vi "Filter and Sort Items.vi"(5 "Sort Info":T5={"Sort Column"=enum."Description", "Ascending?"=FALSE, "Enabled?"=FALSE}, 7 "Filter Info":T7={"Filter Column"=enum."Description", "Filter Type"=enum."Contains", "Filter Value"="", "New Data?"=FALSE, "Enabled?"=FALSE}, 8 "error in (no error)":errorcluster, 10 "New VI Data":T1[](array[typedef]), 11 "Saved VI Data":T1[](array[typedef])) -> (0 "error out":errorcluster, 1 "Displayed Indices":i32[](array[numeric]), 2 "New VI Data out":T1[](array[typedef]), 3 "Saved VI Data out":T1[](array[typedef]))   [LabVIEW 2020, in "VI Properties Editor.lvlib"]
doc: "Filters <B>Saved VI Data</B> according to <B>Filter</B>."
uses:
  VI Properties Editor.lvlib
  <vilib>/regexp/Match Regular Expression.xnode
  <vilib>/picture/picture.llb/imagedata.ctl
  CTLs/VI Properties.ctl
  CTLs/Control Properties.ctl
  CTLs/VI Data.ctl
  CTLs/Column Name.ctl
  CTLs/Filter Type.ctl
  CTLs/Filter Info.ctl
  CTLs/Sort Info.ctl
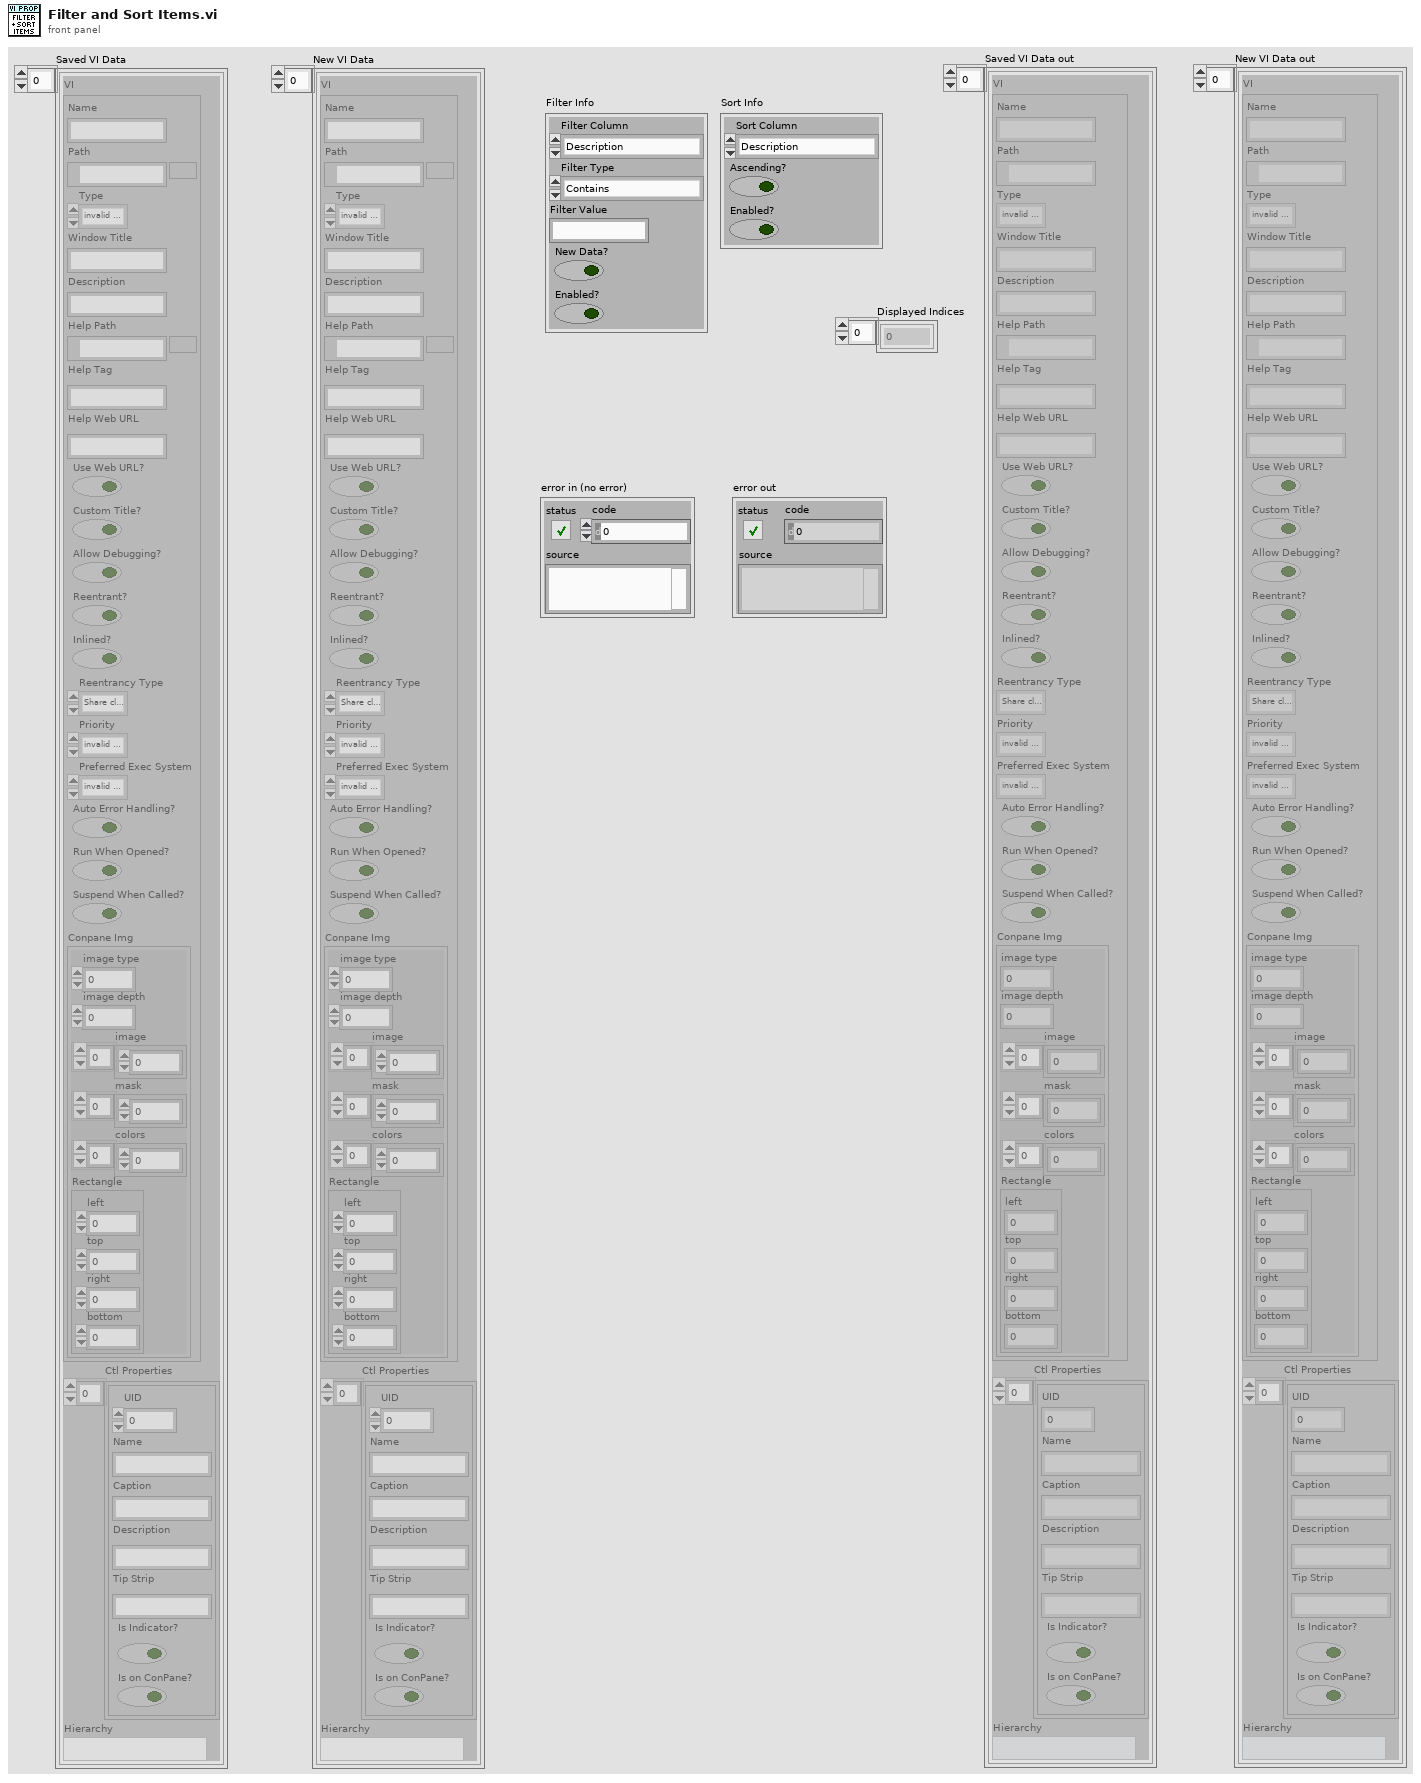
[diagram p1: front panel]
types:
  T1 = typedef "VI Properties Editor.lvlib/VI Data.ctl" = cluster{"VI":T2, "Ctl Properties":T4[], "Hierarchy":string}
  T2 = typedef "VI Properties Editor.lvlib/VI Properties.ctl" = cluster{"Name":string, "Path":path, "Type":enum32{"invalid VI type", "Standard VI", "Control VI", "Global VI", "Polymorphic VI", "Configuration VI", "SubSystem", "Facade VI", "Method VI", "Statechart Diagram VI"}, "Window Title":string, "Description":string, "Help Path":path, "Help Tag":string, "Help Web URL":string, "Use Web URL?":bool, "Custom Title?":bool, "Allow Debugging?":bool, "Reentrant?":bool, "Inlined?":bool, "Reentrancy Type":enum16{"Share clones between instances", "Preallocate clone for each instance"}, "Priority":enum32{"invalid priority", "background priority", "normal priority", "above normal priority", "high priority", "time critical priority", "subroutine"}, "Preferred Exec System":enum32{"invalid execution system", "user interface", "standard", "instrument i/o", "data acquisition", "other 1", "other 2", "same as caller"}, "Auto Error Handling?":bool, "Run When Opened?":bool, "Suspend When Called?":bool, "Conpane Img":T3}
  T3 = typedef "imagedata.ctl" = cluster{"image type":i32, "image depth":i32, "image":u8[], "mask":u8[], "colors":u32[], "Rectangle":cluster{"left":i16, "top":i16, "right":i16, "bottom":i16}}
  T4 = typedef "VI Properties Editor.lvlib/Control Properties.ctl" = cluster{"UID":i32, "Name":string, "Caption":string, "Description":string, "Tip Strip":string, "Is Indicator?":bool, "Is on ConPane?":bool}
  T5 = typedef "VI Properties Editor.lvlib/Sort Info.ctl" = cluster{"Sort Column":T6, "Ascending?":bool, "Enabled?":bool}
  T6 = typedef "VI Properties Editor.lvlib/Column Name.ctl" = enum16{"Name", "Path", "Type", "Window Title", "Description", "Help Path", "Help Tag", "Custom Title?", "Reentrancy", "Inlined?", "Help URL", "Help Type", "Allow Debugging?", "Auto Error Handling?", "Run When Opened?", "Suspend When Called?", "Priority", "Preferred Exec Sytem"}
  T7 = typedef "VI Properties Editor.lvlib/Filter Info.ctl" = cluster{"Filter Column":T6, "Filter Type":T8, "Filter Value":string, "New Data?":bool, "Enabled?":bool}
  T8 = typedef "VI Properties Editor.lvlib/Filter Type.ctl" = enum16{"Contains", "Equals", "Starts with", "Ends with", "Does not contain", "Does not equal", "Is empty", "Is not empty"}
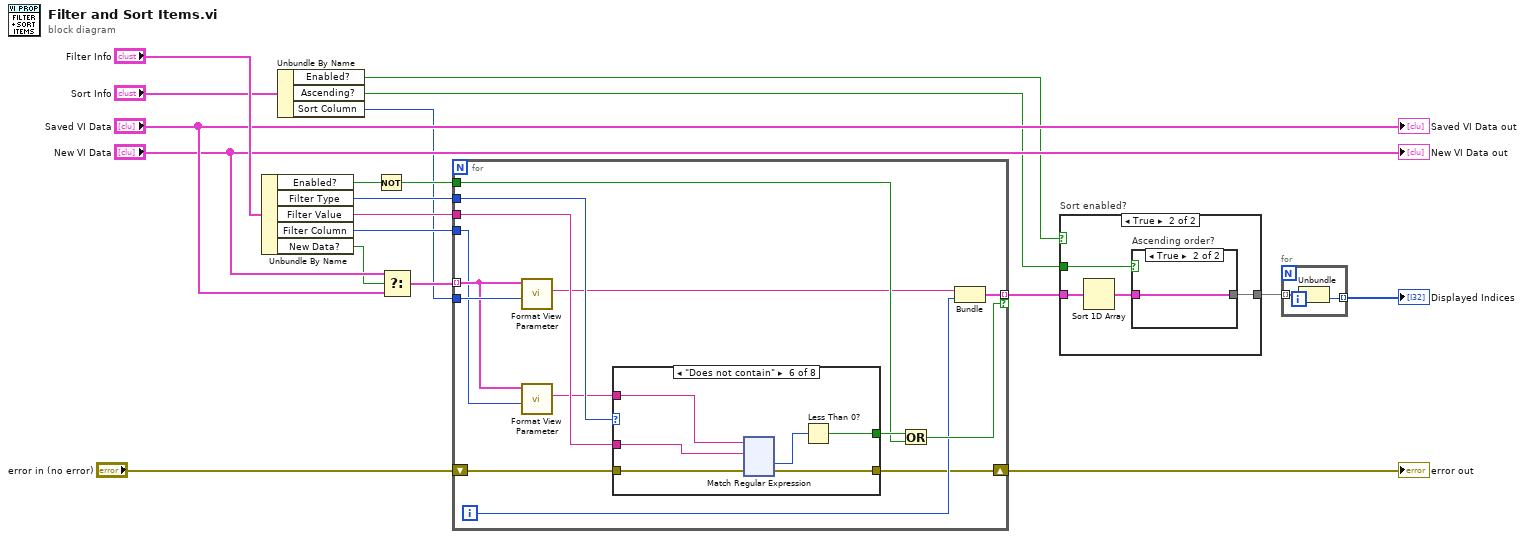
[diagram p0: block diagram]
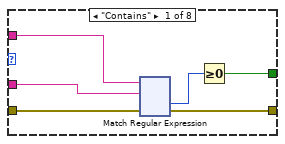
[diagram p2: hidden frame]
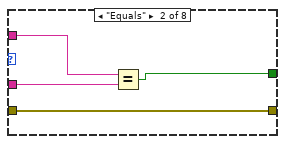
[diagram p3: hidden frame]
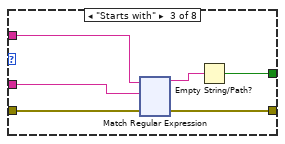
[diagram p4: hidden frame]
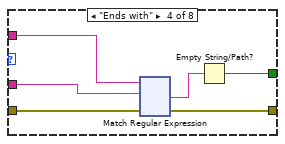
[diagram p5: hidden frame]
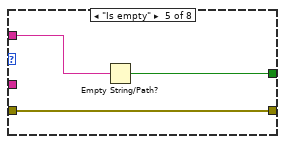
[diagram p6: hidden frame]
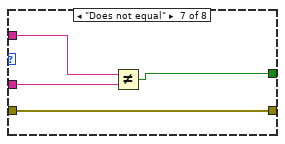
[diagram p7: hidden frame]
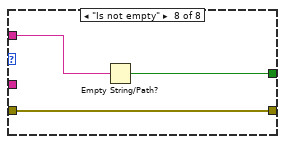
[diagram p8: hidden frame]
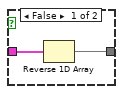
[diagram p10: hidden frame]
diagram:
  n1 = Unbundle By Name("Filter Info") -> ("Enabled?"=w3:bool, "Filter Type"=w18:T8, "Filter Value"=w17:string, "Filter Column"=w5:T6, "New Data?"=w6:bool)
  n2 = Unbundle By Name("Sort Info") -> ("Enabled?"=w1:bool, "Ascending?"=w2:bool, "Sort Column"=w4:T6)
  n3 = Not(x=w3) -> (.not. x?=w16:bool)
  n4 = Select(t="New VI Data", s=w6, f="Saved VI Data") -> (s? t:f=w10:T1[])
  n5 = for {
    tunnel: w10 -> [w22] mode=indexing
    tunnel: w5 -> [w21]
    tunnel: w18 -> [w33]
    tunnel: w17 -> [w32]
    tunnel: [w27] -> w15 mode=indexing if=w30
    tunnel: w16 -> [w29]
    tunnel: w4 -> [w23]
    shift-right: [w25] -> w7
    shift-left: "error in (no error)" -> [w26]
    i -> [w28]
    n6 = call "Format View Parameter.vi"("Column"=w23, "VI Data"=w22) -> ("View Parameter"=w24:string)  [unwired: 9 in]
    n7 = call "Format View Parameter.vi"("Column"=w21, "VI Data"=w22) -> ("View Parameter"=w20:string)  [unwired: 9 in]
    n8 = case shown="\"Does not contain\"" w33 {
      tunnel: w32 -> [w38 w159 w164 w287 _ w414 w535 _]
      tunnel: w20 -> [w39 w160 w166 w289 w409 w415 w536 w539]
      tunnel: [w36 w158 w165 w288 w408 w412 w534 w538] -> w31
      tunnel: w26 -> [w35 w157 w162 w285 w407 w411 w533 w537]
      tunnel: [w34 w157 w161 w284 w407 w410 w533 w537] -> w25
      frame "Contains" {
        n9 = xnode "Match Regular Expression"("input string"=w39, "regular expression"=w38, "error in"=w35) -> ("offset past match"=w37:i32, "error out"=w34:errorcluster)  [unwired: 3 in, 3 out]
        n10 = Greater Or Equal To 0?(x=w37) -> (x >= 0?=w36:bool)
      }
      frame "Equals" {
        n11 = Equal?(x=w160, y=w159) -> (x = y?=w158:bool)
      }
      frame "Starts with" {
        n12 = xnode "Match Regular Expression"("input string"=w166, "regular expression"=w164, "error in"=w162) -> ("before match"=w163:string, "error out"=w161:errorcluster)  [unwired: 3 in, 3 out]
        n13 = Empty String/Path?(string/path=w163) -> (empty?=w165:bool)
      }
      frame "Ends with" {
        n14 = xnode "Match Regular Expression"("input string"=w289, "regular expression"=w287, "error in"=w285) -> ("after match"=w286:string, "error out"=w284:errorcluster)  [unwired: 3 in, 3 out]
        n15 = Empty String/Path?(string/path=w286) -> (empty?=w288:bool)
      }
      frame "Is empty" {
        n16 = Empty String/Path?(string/path=w409) -> (empty?=w408:bool)
      }
      frame "Does not contain" {
        n17 = xnode "Match Regular Expression"("input string"=w415, "regular expression"=w414, "error in"=w411) -> ("offset past match"=w413:i32, "error out"=w410:errorcluster)  [unwired: 3 in, 3 out]
        n18 = Less Than 0?(x=w413) -> (x < 0?=w412:bool)
      }
      frame "Does not equal" {
        n19 = Not Equal?(x=w536, y=w535) -> (x != y?=w534:bool)
      }
      frame "Is not empty" {
        n20 = Empty String/Path?(string/path=w539) -> (empty?=w538:bool)
      }
    }
    n21 = Or(x=w31, y=w29) -> (x .or. y?=w30:bool)
    n22 = Bundle("View Parameter"=w24, w28) -> (w27:cluster{"View Parameter":string, i32})  [unwired: 1 in]
  }
  "error out" <- w7
  n23 = case "Sort enabled?" shown="True" w1 {
    tunnel: w15 -> [w540 w544]
    tunnel: [w540 w542] -> w14
    tunnel: w2 -> [_ w541]
    frame False {
    }
    frame True {
      n24 = Sort 1D Array(array=w544) -> (sorted array=w543:cluster{"View Parameter":string, i32}[])
      n25 = case "Ascending order?" shown="True" w541 {
        tunnel: w543 -> [w546 w547]
        tunnel: [w545 w547] -> w542
        frame False {
          n26 = Reverse 1D Array(array=w546) -> (reversed array=w545:cluster{"View Parameter":string, i32}[])
        }
        frame True {
        }
      }
    }
  }
  n27 = for {
    tunnel: w14 -> [w549] mode=indexing
    tunnel: [w548] -> w13 mode=indexing
    n28 = Unbundle(w549) -> (w548:i32)  [unwired: 1 out]
  }
  "Displayed Indices" <- w13
  "Saved VI Data out" <- "Saved VI Data"
  "New VI Data out" <- "New VI Data"
